vi "ble_discover_ble_devices_170203.vi"(8 "error in (no error)":errorcluster, 9 "LED ref":refnum<vi>, 11 "COM Bluegiga in":refnum<visa-resource-name>) -> (0 "error out":errorcluster, 2 "Devices":string[][](array[string]), 3 "COM Bluegiga out":refnum<visa-resource-name>)   [LabVIEW 2015]
uses:
  type_def/gap_discover_mode.ctl
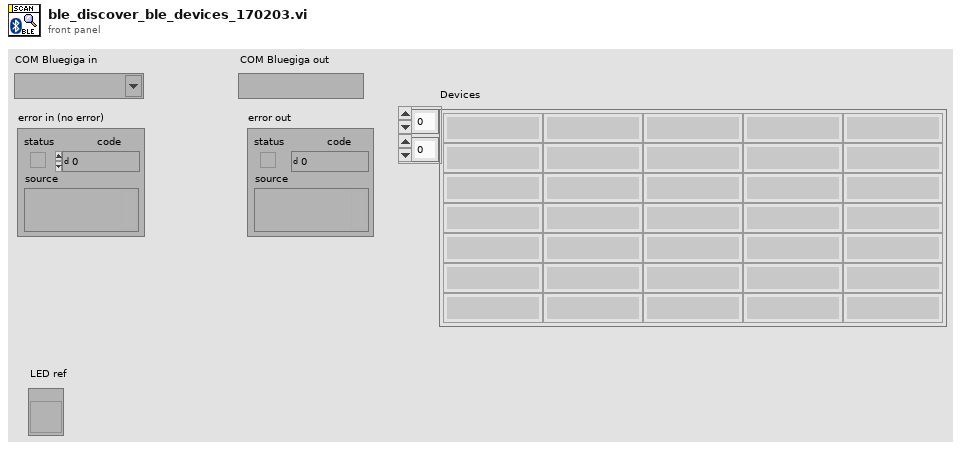
[diagram p1: front panel]
types:
  T1 = typedef "gap_discover_mode.ctl" = u8
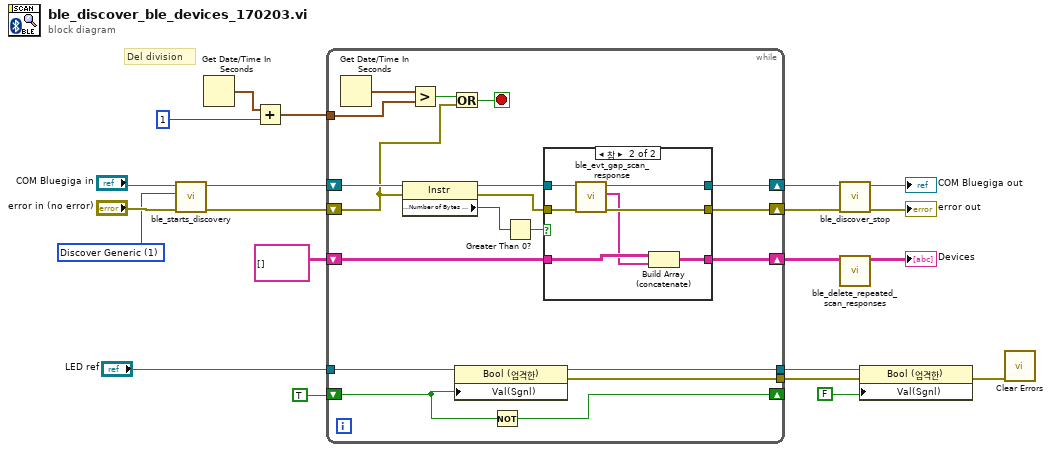
[diagram p0: block diagram]
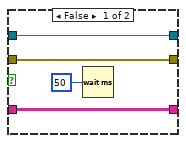
[diagram p2: hidden frame]
diagram:
  w11 = T1 1 items=["Discover Limited", "Discover Generic", "Discover Observation"] ("GAP Discover Mode (Generic)")
  # "Del division"
  n1 = call "ble_starts_discovery.vi"("error in (no error)"="error in (no error)", "GAP Discover Mode (Generic)"=w11, "COM Bluegiga in"="COM Bluegiga in") -> ("error out"=w16:errorcluster, "COM Bluegiga out"=w17:refnum<visa-resource-name>)  [unwired: 5 in, 2 out]
  n2 = Get Date/Time In Seconds() -> (seconds since 1Jan1904=w19:timestamp)
  n3 = Add(x=w19, y=1) -> (x+y=w18:timestamp)
  n4 = while {
    tunnel: w18 -> [w39]
    shift-right: [w33] -> w14
    shift-left: w17 -> [w38]
    shift-right: [w32] -> w15
    shift-left: w16 -> [w27]
    shift-right: [w28] -> w9
    shift-left: string[][] [] -> [w29]
    tunnel: [w26] -> w5
    tunnel: "LED ref" -> [w25]
    shift-right: [w23] -> _
    shift-left: TRUE -> [w24]
    tunnel: [w22] -> w4
    stop <- w30 stop-if-true
    n5 = Get Date/Time In Seconds() -> (seconds since 1Jan1904=w40:timestamp)
    n6 = property class="Instr"(reference=w38, error in=w27) -> (reference out=w36:refnum<visa-resource-name>, error out=w35:errorcluster, "Serial Settings:Number of Bytes at Serial Port"=w37:u32)
    n7 = Greater?(x=w40, y=w39) -> (0:w31:bool)
    n8 = Or(x=w31, y=w27) -> (x .or. y?=w30:bool)
    n9 = property class="Bool (엄격한)"(reference=w25, "Val(Sgnl)"=w24) -> (reference out=w22:refnum<vi>, error out=w26:errorcluster)  [unwired: 1 in]
    n10 = Not(x=w24) -> (.not. x?=w23:bool)
    n11 = Greater Than 0?(x=w37) -> (x > 0?=w34:bool)
    n12 = case shown="참" w34 {
      tunnel: w36 -> [w44 w51]
      tunnel: w35 -> [w43 w48]
      tunnel: [w44 w50] -> w33
      tunnel: [w43 w49] -> w32
      tunnel: w29 -> [w41 w47]
      tunnel: [w41 w45] -> w28
      frame False {
        n13 = Wait (ms)(milliseconds to wait=u32 50) -> ()  [unwired: 1 out]
      }
      frame True {
        n14 = call "ble_evt_gap_scan_response.vi"("error in (no error)"=w48, "COM Bluegiga in"=w51) -> ("error out"=w49:errorcluster, "Scan Response 1 Device"=w46:string[], "COM Bluegiga out"=w50:refnum<visa-resource-name>)  [unwired: 7 in]
        n15 = Build Array (concatenate)(w47, w46) -> (w45:string[][])
      }
    }
  }
  n16 = call "ble_discover_stop.vi"("error in (no error)"=w15, "COM Bluegiga in"=w14) -> ("error out"=→"error out":errorcluster, "COM Bluegiga out"=→"COM Bluegiga out":refnum<visa-resource-name>)  [unwired: 6 in, 2 out]
  n17 = call "ble_delete_repeated_scan_responses.vi"("Scan Responses"=w9) -> ("Unique Scan Responses"=→"Devices":string[][])  [unwired: 10 in]
  n18 = property class="Bool (엄격한)"(reference=w4, error in=w5, "Val(Sgnl)"=FALSE) -> (error out=w3:errorcluster)  [unwired: 1 out]
  n19 = call <vilib>:"Clear Errors.vi"("error in (no error)"=w3) -> ()  [unwired: 5 in, 2 out]
